vi "Get Charact Data By Type.vi"(0 "Charact Data":T2[](array[typedef]), 5 "Standard Type":T1) -> (4 "Found":bool, 6 "Frequencies":dbl[](array[numeric]), 8 "S11":cdb[](array[numeric]))   [LabVIEW 2023, in "RFFixtureCharact.Instruments.lvlib" / "Cal Standard Base.lvclass"]
uses:
  Cal Standard Base.lvclass
  Type Definitions/One-Port Charact Data.ctl
  Type Definitions/Standard Type.ctl
  RFFixtureCharact.Instruments.lvlib
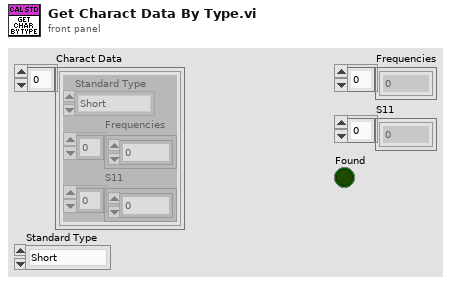
[diagram p1: front panel]
types:
  T1 = typedef "RFFixtureCharact.Instruments.lvlib/Standard Type.ctl" = enum16{"Short", "Open", "Load"}
  T2 = typedef "RFFixtureCharact.Instruments.lvlib/One-Port Charact Data.ctl" = cluster{"Standard Type":T1, "Frequencies":dbl[], "S11":cdb[]}
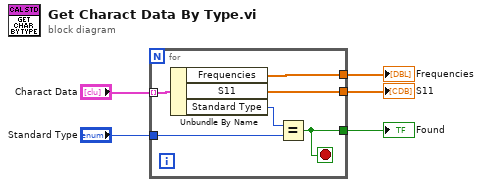
[diagram p0: block diagram]
diagram:
  n1 = for {
    tunnel: "Charact Data" -> [w11] mode=indexing
    tunnel: "Standard Type" -> [w10]
    tunnel: [w8] -> w3
    tunnel: [w7] -> w2
    tunnel: [w6] -> w1
    stop <- w6 stop-if-true
    n2 = Unbundle By Name(w11) -> ("Frequencies"=w8:dbl[], "S11"=w7:cdb[], "Standard Type"=w9:T1)
    n3 = Equal?(x=w9, y=w10) -> (x = y?=w6:bool)
  }
  "Frequencies" <- w3
  "S11" <- w2
  "Found" <- w1
